vi "new.vi"(0 "HGF_Factory":refnum<class "HGF_Factory.lvclass">, 1 "objectName":string, 3 "initializationData":variant, 5 "error in (no error)":errorcluster, 6 "className":string, 7 "binaryString":string, 8 "I8 Array":i8[](array[numeric]), 9 "prependSize? (T)":bool=TRUE, 11 "byteOrder (0:big-endian":T1(ring)) -> (14 "objectRef":refnum<class "HGF_Reference.lvclass">, 17 "found?":bool, 19 "error out":errorcluster)   [LabVIEW 2012, in "HGF_ObjectManager.lvlib"]
doc: "Create and initialize a new object and add it to the global Object Manager database."
uses:
  HGF_ObjectManager.lvlib
  HGF_BaseClasses/HGF_Factory/HGF_Factory.lvclass
  HGF_BaseClasses/HGF_Reference/HGF_Reference.lvclass
  action.ctl
  HGF_Auxiliary/ErrorCode.ctl
  HGF_Auxiliary/Severity.ctl
  HGF_Auxiliary/HGF_Auxiliary.lvlib
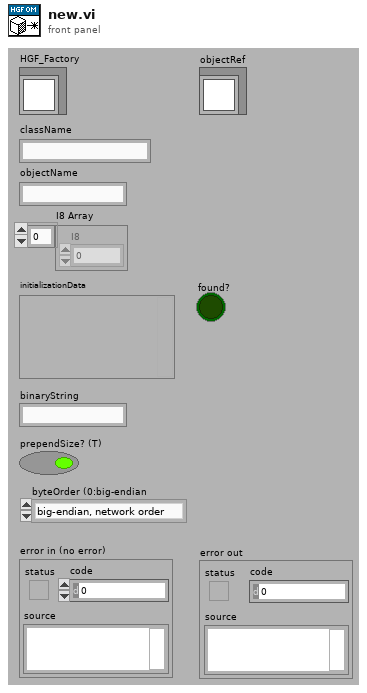
[diagram p1: front panel]
types:
  T1 = enum16{"big-endian, network order", "native, host order", "little-endian"}
  T2 = typedef "HGF_ObjectManager.lvlib/action.ctl" = enum16{"add", "remove", "name2ref", "ref2name ", "obj exists?", "cleanup", "get object list", "reset"}
  T3 = typedef "HGF_Auxiliary.lvlib/Severity.ctl" = enum16{"Info", "Warning", "Fault", "Error", "Fatal"}
  T4 = typedef "HGF_Auxiliary.lvlib/ErrorCode.ctl" = enum32{"No error", "Function not supported.", "This VI is for friends only.", "Reference object aready exisits.", "Parameter out of range.", "Not a rendezvous.", "Invalid notifier reference.", "Invalid queue reference.", "Self-Test not supported.", "Reset not supported.", "IDN query not supported.", "Error query not supported.", "Incorrect addressee.", "Object already exists.", "No class name specified", "Driver not supported", "Attribute is not writable"}
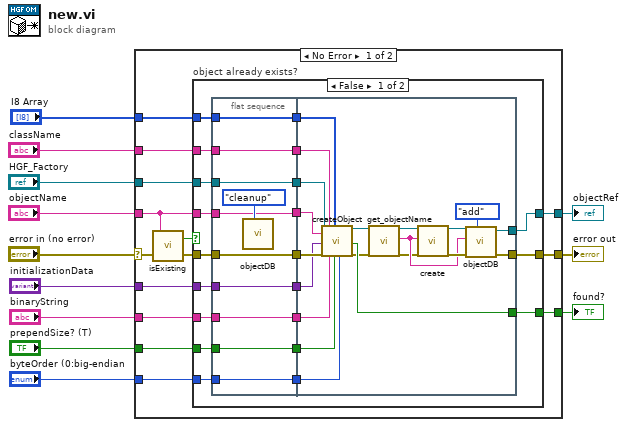
[diagram p0: block diagram]
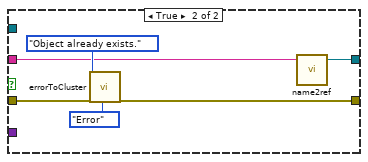
[diagram p2: hidden frame]
diagram:
  n1 = case shown="No Error" "error in (no error)" {
    selector: "error in (no error)" -> [w14 w84]
    tunnel: "objectName" -> [w25 _]
    tunnel: [w23 w84] -> w11
    tunnel: "HGF_Factory" -> [w22 _]
    tunnel: "className" -> [w21 _]
    tunnel: "initializationData" -> [w20 _]
    tunnel: "I8 Array" -> [w19 _]
    tunnel: "binaryString" -> [w18 _]
    tunnel: "prependSize? (T)" -> [w17 _]
    tunnel: "byteOrder (0:big-endian" -> [w16 _]
    tunnel: [w15 _] -> w3
    tunnel: [w13 _] -> w1
    frame No Error {
      n2 = call "isExisting.vi"("error in (no error)"=w14, "name"=w25) -> ("error out"=w24:errorcluster, "obj exists"=w26:bool)
      n3 = case "object already exists?" shown="False" w26 {
        tunnel: w25 -> [w46 w79]
        tunnel: w24 -> [w47 w83]
        tunnel: [w29 w80] -> w23
        tunnel: w22 -> [w42 _]
        tunnel: w21 -> [w41 _]
        tunnel: w20 -> [w38 _]
        tunnel: w19 -> [w36 _]
        tunnel: w18 -> [w34 _]
        tunnel: w17 -> [w32 _]
        tunnel: w16 -> [w30 _]
        tunnel: [w28 w78] -> w15
        tunnel: [w27 _] -> w13
        frame False {
          n4 = flat-sequence {
            tunnel: w47 -> [w56]
            tunnel: w46 -> [w55]
            tunnel: [w56] -> w45
            tunnel: [w55] -> w44
            tunnel: [w54] -> w43
            tunnel: w42 -> [w54]
            tunnel: w41 -> [w53]
            tunnel: [w53] -> w40
            tunnel: [w52] -> w39
            tunnel: w38 -> [w52]
            tunnel: [w51] -> w37
            tunnel: w36 -> [w51]
            tunnel: [w50] -> w35
            tunnel: w34 -> [w50]
            tunnel: [w49] -> w33
            tunnel: w32 -> [w49]
            tunnel: [w48] -> w31
            tunnel: w30 -> [w48]
            tunnel: w45 -> [w77]
            tunnel: w44 -> [w63]
            tunnel: w43 -> [w76]
            tunnel: w40 -> [w75]
            tunnel: w39 -> [w71]
            tunnel: w37 -> [w70]
            tunnel: w35 -> [w69]
            tunnel: w33 -> [w68]
            tunnel: w31 -> [w67]
            tunnel: [w66] -> w29
            tunnel: [w65] -> w28
            tunnel: [w64] -> w27
            frame #0 {
              n5 = call "objectDB.vi"("Action"=action."cleanup") -> ()  [unwired: 4 in, 7 out]
            }
            frame #1 {
              n6 = call "createObject.vi"("HGF_Factory"=w76, "objectName"=w63, "initializationData"=w71, "error in (no error)"=w77, "className"=w75, "binaryString"=w69, "I8 Array"=w70, "prependSize? (T)"=w68, "byteOrder (0:big-endian, network order)"=w67) -> ("HGF_Object"=w62:refnum<class "HGF_Factory.lvclass">, "found?"=w64:bool, "error out"=w59:errorcluster)  [unwired: 8 out]
              n7 = call "get_objectName.vi"("HGF_Factory"=w62, "error in (no error)"=w59) -> ("dup HGF_Factory"=w61:refnum<class "HGF_Factory.lvclass">, "objectName"=w60:string, "error out"=w58:errorcluster)  [unwired: 15 out]
              n8 = call "create.vi"("Object"=w61, "name"=w60, "error in (no error)"=w58) -> ("HGF_Reference"=w73:refnum<class "HGF_Reference.lvclass">, "error out"=w74:errorcluster)  [unwired: 15 out]
              n9 = call "objectDB.vi"("Action"=action."add", "error in (no error)"=w74, "name"=w60, "objectRef"=w73) -> ("error out"=w66:errorcluster, "objectRef out"=w65:refnum<class "HGF_Reference.lvclass">)  [unwired: 1 in, 5 out]
            }
          }
        }
        frame True {
          n10 = call "errorToCluster.vi"("error code"=ErrorCode."Object already exists.", "error in (no error)"=w83, "severity (Error)"=Severity."Error") -> ("error out"=w80:errorcluster)  [unwired: 2 in, 14 out]
          n11 = call "name2ref.vi"("name"=w79) -> ("objectRef out"=w78:refnum<class "HGF_Reference.lvclass">)  [unwired: 1 in, 3 out]
        }
      }
    }
    frame Error {
    }
  }
  "error out" <- w11
  "objectRef" <- w3
  "found?" <- w1
